vi "tcp_receiver (SubVI).vi"(8 "error in (no error)":errorcluster, 11 "TCP Network Connection in":refnum<k5>) -> (1 "data in string 2":string, 2 "array type (2D Dbl)":dbl[](array[numeric]), 3 "length 2":i32)   [LabVIEW 2015]
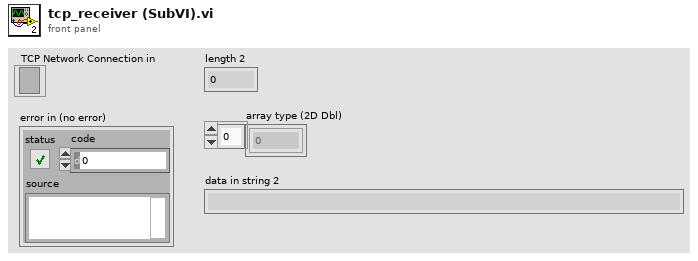
[diagram p1: front panel]
types:
  T1 = enum16{"Standard", "Buffered", "CRLF", "Immediate"}
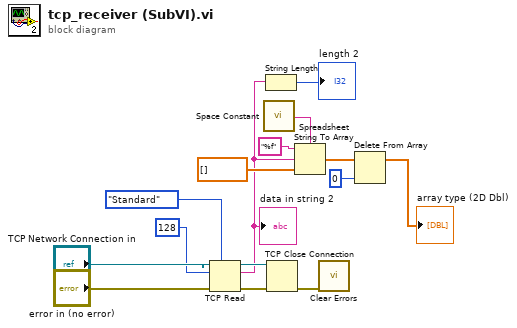
[diagram p0: block diagram]
diagram:
  n1 = TCP Read(connection ID="TCP Network Connection in", bytes to read=128, error in (no error)="error in (no error)", 7:T1."Standard" ("mode (standard)")) -> (connection ID out=w10:refnum<k5>, data out=w4:string, error out=w9:errorcluster)  [unwired: 1 in]
  "data in string 2" <- w4
  n2 = call <vilib>:"Space Constant.vi"() -> ("String"=w12:string)
  n3 = String Length(string=w4) -> (length=→"length 2":i32)
  n4 = TCP Close Connection(connection ID=w10, error in (no error)=w9) -> (error out=w11:errorcluster)  [unwired: 1 in, 1 out]
  n5 = Spreadsheet String To Array(delimiter (Tab)=w12, format string="%f", spreadsheet string=w4, array type (2D Dbl)=dbl[] []) -> (array=w2:dbl[])
  n6 = call <vilib>:"Clear Errors.vi"("error in (no error)"=w11) -> ()  [unwired: 5 in, 2 out]
  n7 = Delete From Array(array=w2, index=0) -> (array with subset deleted=→"array type (2D Dbl)":dbl[])  [unwired: 1 in, 1 out]
